vi "Theta Drive_One step on.vi"(11 "stop":bool) -> (3 "Boolean array":bool[](array[boolean]))   [LabVIEW 2017]
uses:
  <vilib>/myRIO/Instrument Drivers/Onboard IO/DIO/typedefs/DIO Reference.ctl
  <vilib>/myRIO/Common/Instrument Driver Framework/Utilities/typedefs/myRIO Generic Hardware Reference.ctl
  <vilib>/myRIO/Common/Instrument Driver Framework/Utilities/typedefs/Hardware Version Enum.ctl
  <vilib>/myRIO/Common/Instrument Driver Framework/Utilities/typedefs/myRIO v1.0 Reference.ctl
  <vilib>/myRIO/Common/Instrument Driver Framework/Utilities/typedefs/Generic FPGA Reference.ctl
  <vilib>/myRIO/Common/Instrument Driver Framework/myRIO v1.0/DIO/typedefs/DIO Channels List.ctl
  <vilib>/myRIO/Common/Instrument Driver Framework/myRIO v1.0/DIO/typedefs/DIO Channels Enum.ctl
  <vilib>/userdefined/High Color/nirio_resource_hc.ctl
  <vilib>/myRIO/Common/Instrument Driver Framework/Utilities/vis/Is FPGA Ref Available.vi
  <vilib>/myRIO/Common/Instrument Driver Framework/myRIO v1.0/DIO/vis/myRIO v1.1 Open DIO.vi
  <vilib>/myRIO/Instrument Drivers/Onboard IO/DIO/vis/Write.vi
  <vilib>/myRIO/Common/Instrument Driver Framework/Utilities/vis/Validate Channels.vi
  <vilib>/myRIO/Common/Instrument Driver Framework/myRIO v1.0/DIO/vis/myRIO v1.0 Reserve DIO.vi
  <vilib>/myRIO/Common/Instrument Driver Framework/myRIO v1.0/Resource Manager/vis/myRIO v1.0 Reserve Channel List.vi
  <vilib>/myRIO/Common/Instrument Driver Framework/myRIO v1.0/DIO/vis/myRIO v1.0 Build MUX Configuration DIO.vi
  <vilib>/myRIO/Common/Instrument Driver Framework/myRIO v1.0/Resource Manager/vis/myRIO v1.0 Reserve Channel.vi
  <vilib>/myRIO/Common/Instrument Driver Framework/myRIO v1.0/Resource Manager/vis/myRIO v1.0 Unreserve Channel.vi
  <vilib>/myRIO/Common/Instrument Driver Framework/myRIO v1.0/Resource Manager/vis/myRIO v1.0 Create Configuration List.vi
  <vilib>/myRIO/Common/Instrument Driver Framework/myRIO v1.0/Resource Manager/vis/myRIO v1.0 Build Mutex Name.vi
  <vilib>/Utility/VariantDataType/GetNumericInfo.vi
  <vilib>/Utility/error.llb/Error Cluster From Error Code.vi
  <vilib>/myRIO/Common/Instrument Driver Framework/myRIO v1.0/myRIO v1.1 Open.vi
  <vilib>/myRIO/Common/Instrument Driver Framework/Utilities/vis/IO Manager.vi
  <vilib>/myRIO/Common/Instrument Driver Framework/Utilities/vis/Configuration Manager.vi
  <vilib>/myRIO/Common/Instrument Driver Framework/myRIO v1.0/Resource Manager/vis/myRIO v1.0 Configure IO.vi
  <vilib>/myRIO/Common/Instrument Driver Framework/myRIO v1.0/myRIO v1.0 Close.vi
  <vilib>/myRIO/Common/Instrument Driver Framework/myRIO v1.0/DIO/vis/myRIO v1.0 Write DIO.vi
  <vilib>/myRIO/Express VI/Onboard IO/DO/DO Express VI.xnode
  <vilib>/myRIO/Instrument Drivers/Onboard IO/DIO/vis/myRIO DIO Open.xnode
  <vilib>/myRIO/Instrument Drivers/Onboard IO/DIO/DIO.lvlib
panel:
  out "Current Motor Step":i32
  out "Current Step":i32
  in  "Start Location Step (-90to90)":i32
  in  "Target Step (-90to90)":i32
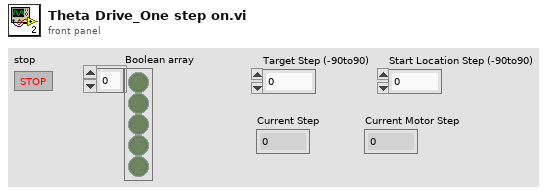
[diagram p1: front panel]
types:
  T1 = typedef "DIO.lvlib/DIO Reference.ctl" = cluster{"myRIO Reference":T2, "DIO Channels List":T6}
  T2 = typedef "myRIO Generic Hardware Reference.ctl" = cluster{"myRIO Model":T3, "myRIO Hardware Reference":T4}
  T3 = typedef "Hardware Version Enum.ctl" = enum16{"Unknown", "myRIO-1900", "myRIO-1950", "roboRIO", "NI ELVIS RIO CM"}
  T4 = typedef "myRIO v1.0 Reference.ctl" = cluster{"Generic FPGA Reference":T5, "Allow multiple opens":bool}
  T5 = typedef "Generic FPGA Reference.ctl" = refnum<k20>
  T6 = typedef "DIO Channels List.ctl" = T7[]
  T7 = typedef "DIO Channels Enum.ctl" = enum16{"Not Connected", "C/DIO0", "C/DIO1", "C/DIO2", "C/DIO3", "C/DIO4", "C/DIO5", "C/DIO6", "C/DIO7", "A/DIO0", "A/DIO1", "A/DIO2", "A/DIO3", "A/DIO4", "A/DIO5", "A/DIO6", "A/DIO7", "A/DIO8", "A/DIO9", "A/DIO10", "A/DIO11", "A/DIO12", "A/DIO13", "A/DIO14", "A/DIO15", "B/DIO0", "B/DIO1", "B/DIO2", "B/DIO3", "B/DIO4", "B/DIO5", "B/DIO6", "B/DIO7", "B/DIO8", "B/DIO9", "B/DIO10", "B/DIO11", "B/DIO12", "B/DIO13", "B/DIO14", "B/DIO15", "LED0", "LED1", "LED2", "LED3", "Button0", "DIO/DIO0", "DIO/DIO1", "DIO/DIO2", "DIO/DIO3", "DIO/DIO4", "DIO/DIO5", "DIO/DIO6", "DIO/DIO7", "DIO/DIO8", "DIO/DIO9", "SPI/CS0", "SPI/CS1", "SPI/CS2", "SPI/CS3", "LED RADIO (Green)", "LED RADIO (Red)", "LED COMM (Green)", "LED COMM (Red)", "LED MODE (Green)", "LED MODE (Red)"}
  T8 = typedef "nirio_resource_hc.ctl" = tag
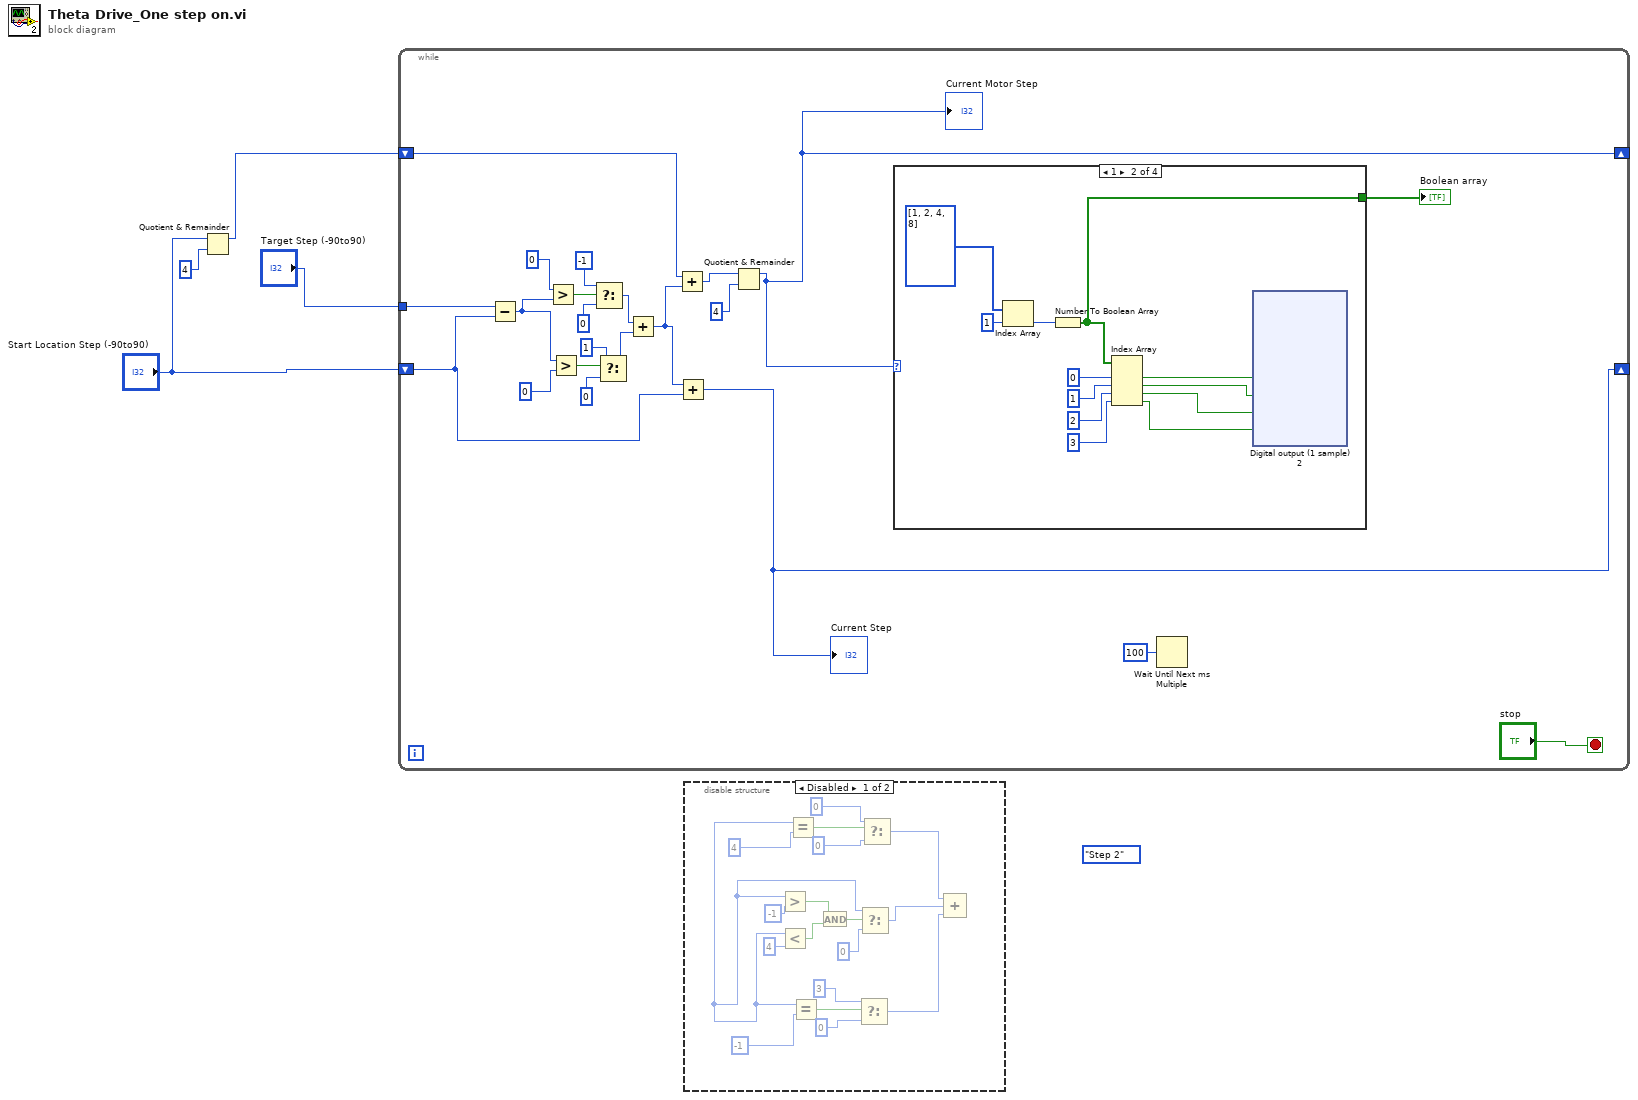
[diagram p0: block diagram]
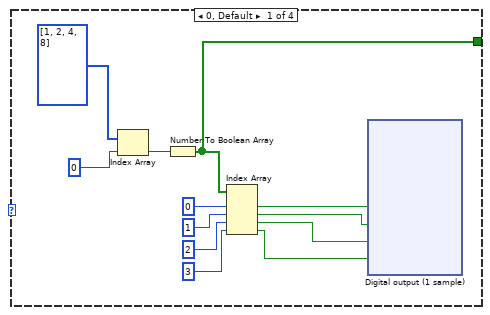
[diagram p3: hidden frame]
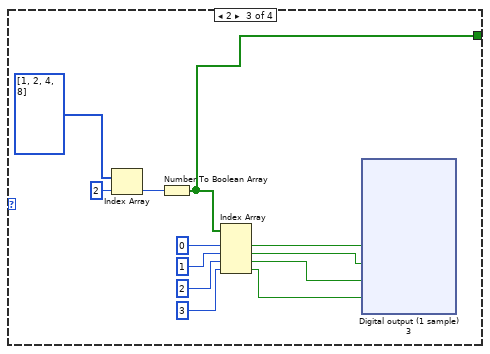
[diagram p4: hidden frame]
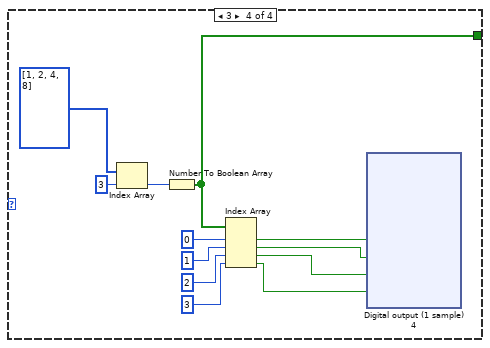
[diagram p5: hidden frame]
diagram:
  (unwired) enum16{"Step 0", "Step 1", "Step 2", "Step 3"}."Step 2"
  n1 = Quotient & Remainder(x="Start Location Step (-90to90)", y=4) -> (x-y*floor(x/y)=w1:i32)  [unwired: 1 out]
  n2 = while {
    shift-right: [w6] -> _
    shift-left: "Start Location Step (-90to90)" -> [w7]
    tunnel: "Target Step (-90to90)" -> [w11]
    shift-right: [w9] -> _
    shift-left: w1 -> [w10]
    stop <- "stop" stop-if-true
    n3 = Subtract(x=w11, y=w7) -> (x-y=w23:i32)
    n4 = Greater?(x=0, y=w23) -> (0:w21:bool)
    n5 = Greater?(x=w23, y=0) -> (0:w18:bool)
    n6 = Select(t=-1, s=w21, f=0) -> (s? t:f=w15:i32)
    n7 = Select(t=1, s=w18, f=0) -> (s? t:f=w14:i32)
    n8 = Add(x=w15, y=w14) -> (x+y=w8:i32)
    n9 = Add(x=w10, y=w8) -> (x+y=w13:i32)
    n10 = Add(x=w8, y=w7) -> (x+y=w6:i32)
    "Current Step" <- w6
    n11 = Quotient & Remainder(x=w13, y=4) -> (x-y*floor(x/y)=w9:i32)  [unwired: 1 out]
    "Current Motor Step" <- w9
    n12 = case shown="1" w9 {
      tunnel: [w30 w79 w128 w178] -> w26
      frame 0, Default {
        n13 = Index Array(array=i32[] [1, 2, 4, 8], index=0) -> (element=w29:i32)
        n14 = Number To Boolean Array(number=w29) -> (Boolean array=w30:bool[])
        n15 = Index Array(array=w30, index #1=0 ("index"), index #2=1 ("index"), index #3=2 ("index"), index #4=3 ("index")) -> (element #1=w38:bool, element #2=w37:bool, element #3=w36:bool, element #4=w35:bool)
        n16 = xnode "Digital output (1 sample)"("A/DIO0 (Pin 11)"=w38, "A/DIO1 (Pin 13)"=w37, "A/DIO2 (Pin 15)"=w36, "A/DIO3 (Pin 17)"=w35) -> ()  [unwired: 1 in, 1 out]
      }
      frame 1 {
        n17 = Index Array(array=i32[] [1, 2, 4, 8], index=1) -> (element=w80:i32)
        n18 = Number To Boolean Array(number=w80) -> (Boolean array=w79:bool[])
        n19 = Index Array(array=w79, index #1=0 ("index"), index #2=1 ("index"), index #3=2 ("index"), index #4=3 ("index")) -> (element #1=w88:bool, element #2=w87:bool, element #3=w86:bool, element #4=w85:bool)
        n20 = xnode "Digital output (1 sample) 2"("A/DIO0 (Pin 11)"=w88, "A/DIO1 (Pin 13)"=w87, "A/DIO2 (Pin 15)"=w86, "A/DIO3 (Pin 17)"=w85) -> ()  [unwired: 1 in, 1 out]
      }
      frame 2 {
        n21 = Index Array(array=i32[] [1, 2, 4, 8], index=2) -> (element=w130:i32)
        n22 = Number To Boolean Array(number=w130) -> (Boolean array=w128:bool[])
        n23 = Index Array(array=w128, index #1=0 ("index"), index #2=1 ("index"), index #3=2 ("index"), index #4=3 ("index")) -> (element #1=w138:bool, element #2=w137:bool, element #3=w136:bool, element #4=w135:bool)
        n24 = xnode "Digital output (1 sample) 3"("A/DIO0 (Pin 11)"=w138, "A/DIO1 (Pin 13)"=w137, "A/DIO2 (Pin 15)"=w136, "A/DIO3 (Pin 17)"=w135) -> ()  [unwired: 1 in, 1 out]
      }
      frame 3 {
        n25 = Index Array(array=i32[] [1, 2, 4, 8], index=3) -> (element=w180:i32)
        n26 = Number To Boolean Array(number=w180) -> (Boolean array=w178:bool[])
        n27 = Index Array(array=w178, index #1=0 ("index"), index #2=1 ("index"), index #3=2 ("index"), index #4=3 ("index")) -> (element #1=w188:bool, element #2=w187:bool, element #3=w186:bool, element #4=w185:bool)
        n28 = xnode "Digital output (1 sample) 4"("A/DIO0 (Pin 11)"=w188, "A/DIO1 (Pin 13)"=w187, "A/DIO2 (Pin 15)"=w186, "A/DIO3 (Pin 17)"=w185) -> ()  [unwired: 1 in, 1 out]
      }
    }
    "Boolean array" <- w26
    n29 = Wait Until Next ms Multiple(millisecond multiple=u32 100) -> ()  [unwired: 1 out]
  }
  n30 = disable-structure shown="Disabled" {
    frame Disabled {
      n31 = Equal?(y=-1) -> (x=w241:i32, x = y?=w236:bool)
      n32 = Greater?(x=w241, y=-1) -> (0:w237:bool)
      n33 = Less?(x=w241, y=4) -> (x < y?=w238:bool)
      n34 = Equal?(x=w241, y=4) -> (x = y?=w240:bool)
      n35 = And(x=w237, y=w238) -> (x .and. y?=w239:bool)
      n36 = Select(t=3, s=w236, f=0) -> (s? t:f=w244:i32)
      n37 = Select(t=w241, s=w239, f=0) -> (s? t:f=w243:i32)
      n38 = Select(t=0, s=w240, f=0) -> (s? t:f=w242:i32)
      n39 = Compound Arithmetic op=ADD(w242, w243, w244) -> ()  [unwired: 1 out]
    }
    frame Enabled {
    }
  }
